vi "Test Unzip Read-Only File.vi"() -> ()   [LabVIEW 2019]
uses:
  <vilib>/addons/_JKI Toolkits/Caraya/classes/Assert/Assert True.vi
  source/Command-Line Zip.lvlib
  <vilib>/addons/_JKI Toolkits/Caraya/classes/Test/Test.lvclass
  <vilib>/addons/_JKI Toolkits/Caraya/classes/Assert/Assert.lvclass
panel:
  out "temp folder location":path
  out "success?":bool
  in  "Delete Temp Folder on Success?":bool=TRUE
  in  "error in":errorcluster
  out "error out":errorcluster
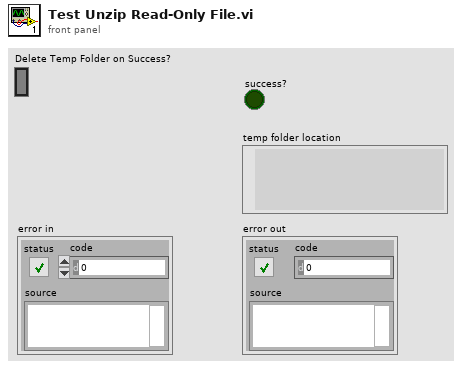
[diagram p1: front panel]
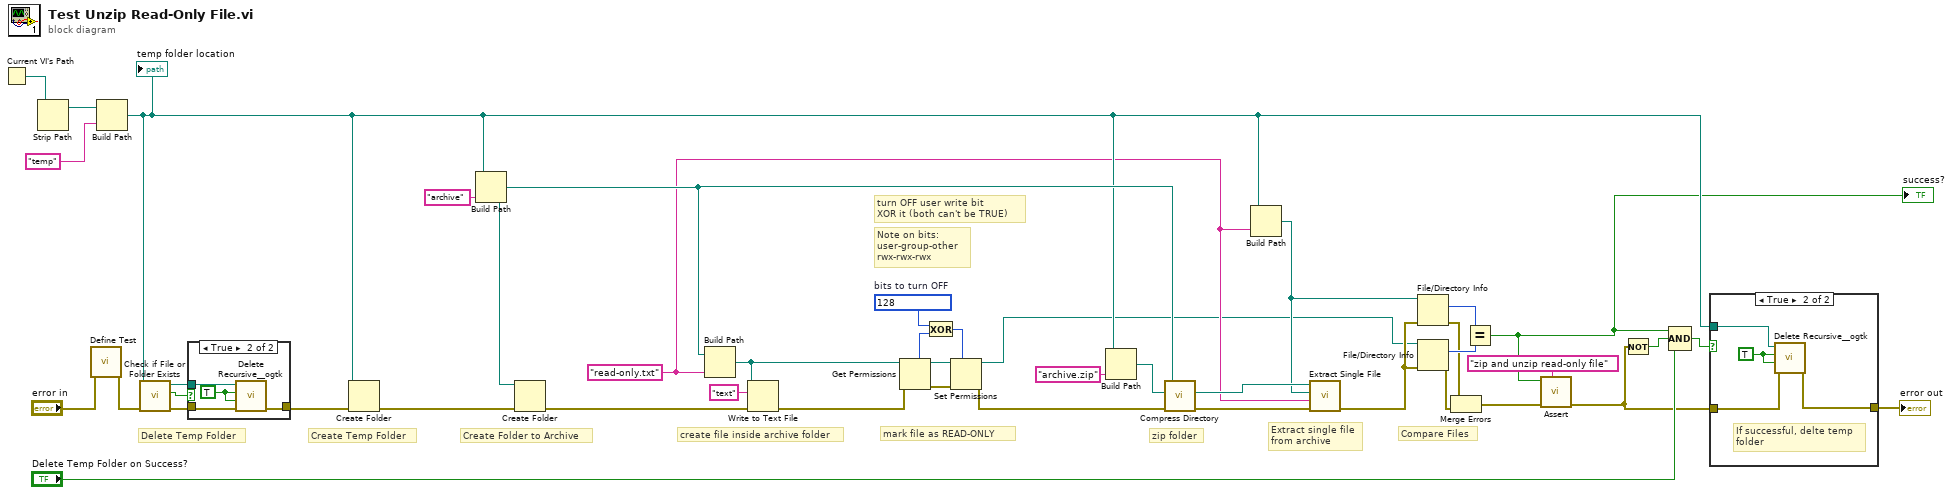
[diagram p0: block diagram]
diagram:
  w6 = i16 128  # bits to turn OFF
  w2 = "read-only.txt" ("name or relative path")
  # "mark file as READ-ONLY"
  # "Note on bits:\nuser-group-other\nrwx-rwx-rwx"
  # "turn OFF user write bit\nXOR it (both can't be TRUE)"
  # "Extract single file from archive"
  # "Compare Files"
  # "zip folder"
  # "create file inside archive folder"
  # "Create Folder to Archive"
  # "Create Temp Folder"
  # "Delete Temp Folder"
  n1 = Current VI's Path() -> (path=w43:path)
  n2 = Strip Path(path=w43) -> (stripped path=w42:path)  [unwired: 1 out]
  n3 = call <vilib>:"Define Test.vi"("error in (no error)"="error in") -> ("error out"=w15:errorcluster)  [unwired: 10 in]
  n4 = Build Path(base path=w42, name or relative path="temp") -> (appended path=w23:path)
  "temp folder location" <- w23
  n5 = call <vilib>:"Check if File or Folder Exists.vi"("error in (no error)"=w15, "path"=w23) -> ("error out"=w30:errorcluster, "file or folder exists?"=w27:bool, "dup path"=w28:path)  [unwired: 7 in]
  n6 = case shown="True" w27 {
    tunnel: w30 -> [w44 w47]
    tunnel: [w44 w48] -> w29
    tunnel: w28 -> [_ w46]
    frame False {
    }
    frame True {
      w45 = TRUE ("Recursive? (FALSE)")
      n7 = call <userlib>:"Delete Recursive__ogtk.vi"("error in (no error)"=w47, "Ignore Read-Only? (FALSE)"=w45, "Recursive? (FALSE)"=w45, "Path"=w46) -> ("error out"=w48:errorcluster)  [unwired: 6 in, 1 out]
    }
  }
  n8 = Create Folder(path (use dialog)=w23, error in=w29) -> (error out=w40:errorcluster)  [unwired: 1 in, 2 out]
  n9 = Build Path(base path=w23, name or relative path="archive") -> (appended path=w24:path)
  n10 = Create Folder(path (use dialog)=w24, error in=w40) -> (error out=w38:errorcluster)  [unwired: 1 in, 2 out]
  n11 = Build Path(base path=w24, name or relative path=w2) -> (appended path=w8:path)
  n12 = Write to Text File(file (use dialog)=w8, text="text", error in=w38) -> (error out=w4:errorcluster)  [unwired: 1 in, 2 out]
  n13 = Get Permissions(8:w4, 11:w8) -> (0:w10:errorcluster, 3:w9:path, 5:w7:i16)  [unwired: 2 out]
  n14 = Exclusive Or(1:w7, 2:w6) -> (0:w5:i16)
  n15 = Set Permissions(7:w5, 8:w10, 11:w9) -> (0:w3:errorcluster, 3:w1:path)  [unwired: 2 in]
  n16 = Build Path(base path=w23, name or relative path="archive.zip") -> (appended path=w34:path)
  n17 = call "Compress Directory.vi"("error in (no error)"=w3, "archive name (root directory with .zip ending)"=w34, "root directory (file dialog)"=w24) -> ("error out"=w36:errorcluster, "archive name out"=w25:path)  [unwired: 6 in, 1 out]
  n18 = Build Path(base path=w23, name or relative path=w2) -> (appended path=w22:path)
  n19 = call "Extract Single File.vi"("error in (no error)"=w36, "name or relative path (\"\": use output file name)"=w2, "File output Path (extract to temp file)"=w22, "Zip File Path"=w25) -> ("error out"=w21:errorcluster)  [unwired: 4 in, 3 out]
  n20 = File/Directory Info(path=w22, error in=w21) -> (size=w20:i64, error out=w18:errorcluster)  [unwired: 5 out]
  n21 = File/Directory Info(path=w1, error in=w21) -> (size=w19:i64, error out=w17:errorcluster)  [unwired: 5 out]
  n22 = Merge Errors(w18, w17) -> (w14:errorcluster)
  n23 = Equal?(x=w20, y=w19) -> (x = y?=w12:bool)
  "success?" <- w12
  n24 = call-poly <vilib>:"Assert.vi"("Label"="zip and unzip read-only file", "error in (no error)"=w14, "True?"=w12) -> ("error out"=w13:errorcluster)  [unwired: 8 in]
  n25 = Not(x=w13) -> (.not. x?=w31:bool)
  n26 = Compound Arithmetic op=AND(w12, w31, "Delete Temp Folder on Success?") -> (w32:bool)
  n27 = case shown="True" w32 {
    tunnel: [w49 w52] -> w33
    tunnel: w13 -> [w49 w51]
    tunnel: w23 -> [_ w50]
    frame False {
    }
    frame True {
      w53 = TRUE ("Recursive? (FALSE)")
      # "If successful, delte temp folder"
      n28 = call <userlib>:"Delete Recursive__ogtk.vi"("error in (no error)"=w51, "Ignore Read-Only? (FALSE)"=w53, "Recursive? (FALSE)"=w53, "Path"=w50) -> ("error out"=w52:errorcluster)  [unwired: 6 in, 1 out]
    }
  }
  "error out" <- w33
